vi "Build String.vi"(7 "conversion blocks":T1[](array[typedef]) {"string offset" format="%d bytes"; "engine offset" format="%d bytes"}, 8 "error in (no error)":errorcluster, 10 "string buffer in":u8[](array[numeric]), 11 "engine buffer in":u8[](array[numeric])) -> (0 "error out":errorcluster, 2 "string buffer out":u8[](array[numeric]), 3 "engine buffer out":u8[](array[numeric]))   [LabVIEW 2017, in "DSF Core.lvlib" / "Default Buffer Converter.lvclass"]
uses:
  Default Buffer Converter.lvclass
  Conversion Block.ctl
  Typedefs/DSF Data Type.ctl
  Classes/Buffer Converter/Convert String Data Type.vi
  VIs/Sizeof 1D.vi
  DSF Core.lvlib
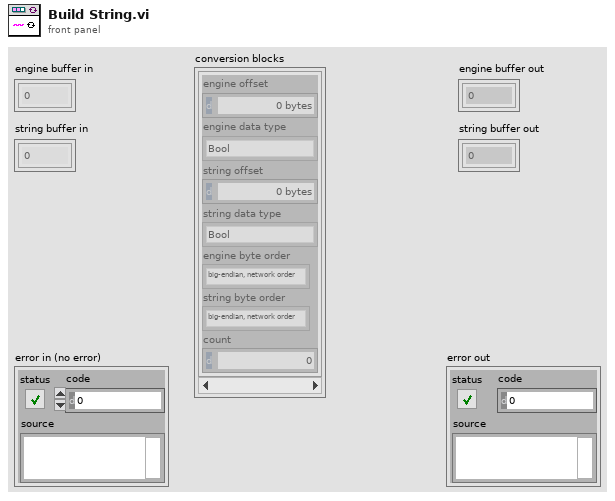
[diagram p1: front panel]
types:
  T1 = typedef "DSF Core.lvlib/Default Buffer Converter.lvclass/Conversion Block.ctl" = cluster{"engine offset":u64, "engine data type":T2, "string offset":u64, "string data type":T2, "engine byte order":enum16{"big-endian, network order", "native, host order", "little-endian"}, "string byte order":enum16{"big-endian, network order", "native, host order", "little-endian"}, "count":u64}
  T2 = typedef "DSF Core.lvlib/DSF Data Type.ctl" = enum8{"Bool", "SGL", "DBL", "I8", "I16", "I32", "I64", "U8", "U16", "U32", "U64"}
  T3 = enum16{"big-endian, network order", "native, host order", "little-endian"}
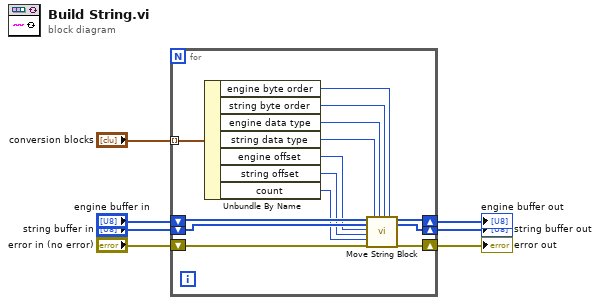
[diagram p0: block diagram]
diagram:
  n1 = for {
    tunnel: "conversion blocks" -> [w20] mode=indexing
    shift-right: [w19] -> w3
    shift-left: "error in (no error)" -> [w21]
    shift-right: [w17] -> w7
    shift-left: "string buffer in" -> [w18]
    shift-right: [w16] -> w6
    shift-left: "engine buffer in" -> [w15]
    n2 = Unbundle By Name(w20) -> ("engine byte order"=w14:T3, "string byte order"=w13:T3, "engine data type"=w12:T2, "string data type"=w11:T2, "engine offset"=w9:u64, "string offset"=w10:u64, "count"=w8:u64)
    n3 = call "Move String Block.vi"("src buffer in"=w15, "dst buffer in"=w18, "src buffer offset"=w9, "dst buffer offset"=w10, "channel count"=w8, "error in (no error)"=w21, "dst data type"=w11, "src data type"=w12, "dst byte order"=w13, "src byte order"=w14) -> ("src buffer out"=w16:u8[], "dst buffer out"=w17:u8[], "error out"=w19:errorcluster)  [unwired: 7 in]
  }
  "engine buffer out" <- w6
  "string buffer out" <- w7
  "error out" <- w3
